vi "Destroy Queue.vi"(8 "error in (no error)":errorcluster) -> (0 "error out":errorcluster, 2 "No. Of Remaining Elements":i32, 3 "Remaining Elements":T1[](array[typedef]))   [LabVIEW 2022 SP3]
doc: "Destroys (or releases) the queue. (Force Destroy is set to TRUE.)"
uses:
  Message.ctl
  Command.ctl
panel:
  # "Development\ncontrols/indicators useful for development and testing, but which are not outputs of the VI"
  # "Input\nInputs to the VI"
  # "Output\nOutputs of the VI"
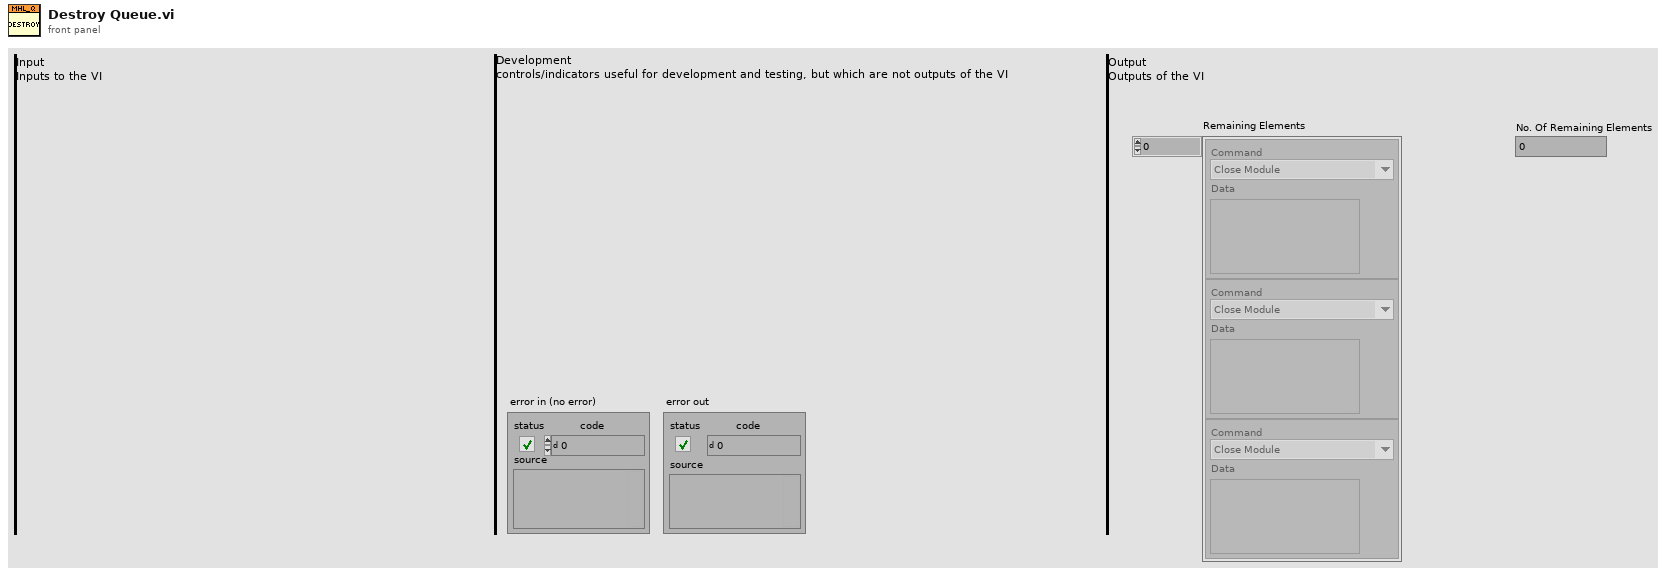
[diagram p1: front panel]
types:
  T1 = typedef "Message.ctl" = cluster{"Command":T2, "Data":variant}
  T2 = typedef "Command.ctl" = enum16{"Init Module", "Close Module", "Local Error Handler", "Init Tickboxes", "Command 2 (replace me)", "Command 3 (replace me)"}
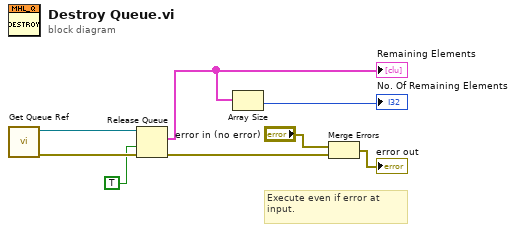
[diagram p0: block diagram]
diagram:
  # "Execute even if error at input."
  n1 = call "Get Queue Ref.vi"() -> ("error out"=w8:errorcluster, "Queue Ref"=w6:refnum<queue>)  [unwired: 10 in]
  n2 = Release Queue(queue=w6, force destroy? (F)=TRUE, error in (no error)=w8) -> (remaining elements=w2:T1[], error out=w7:errorcluster)  [unwired: 1 out]
  "Remaining Elements" <- w2
  n3 = Array Size(array=w2) -> (size(s)=→"No. Of Remaining Elements":i32)
  n4 = Merge Errors("error in (no error)", w7) -> (→"error out":errorcluster)
